vi "Get_DeviceInformation.vi"(8 "error in (no error)":errorcluster, 11 "Abstract_CCD in":refnum<class "Abstract_CCD.lvclass">) -> (0 "error out":errorcluster, 2 "Array":string[](array[string]), 3 "Abstract_CCD out":refnum<class "Abstract_CCD.lvclass">)   [LabVIEW 2020, in "Abstract_CCD.lvclass"]
uses:
  <instrlib>/Classes/CCD/Abstract_CCD/Abstract_CCD.lvclass
  <instrlib>/Classes/CCD/Abstract_CCD/FrameCombination.ctl
panel:
  out "FrameCombinationMethod":T1 items=["Sum"=1, "Average"=2]
  in  "Enum":enum16{"Not Defined", "Unlocked", "Locked"}(ring)
  in  "Trigger Mode":u16(ring) items=["Intern", "Extern"]
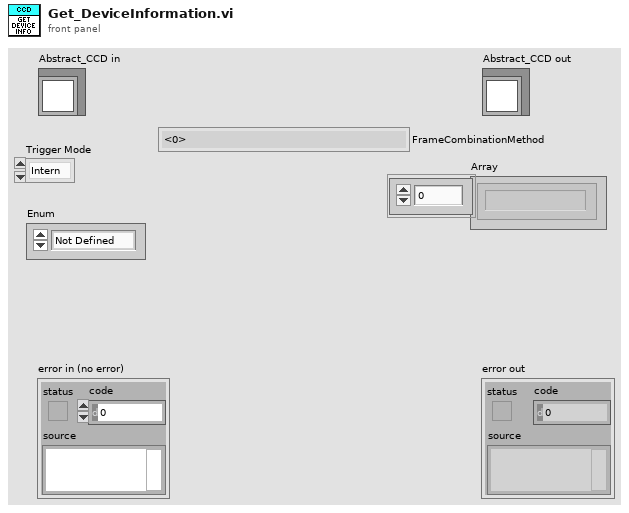
[diagram p1: front panel]
types:
  T1 = typedef "FrameCombination.ctl" = i32
  T2 = enum16{"Not Defined", "Unlocked", "Locked", "Not Reached"}
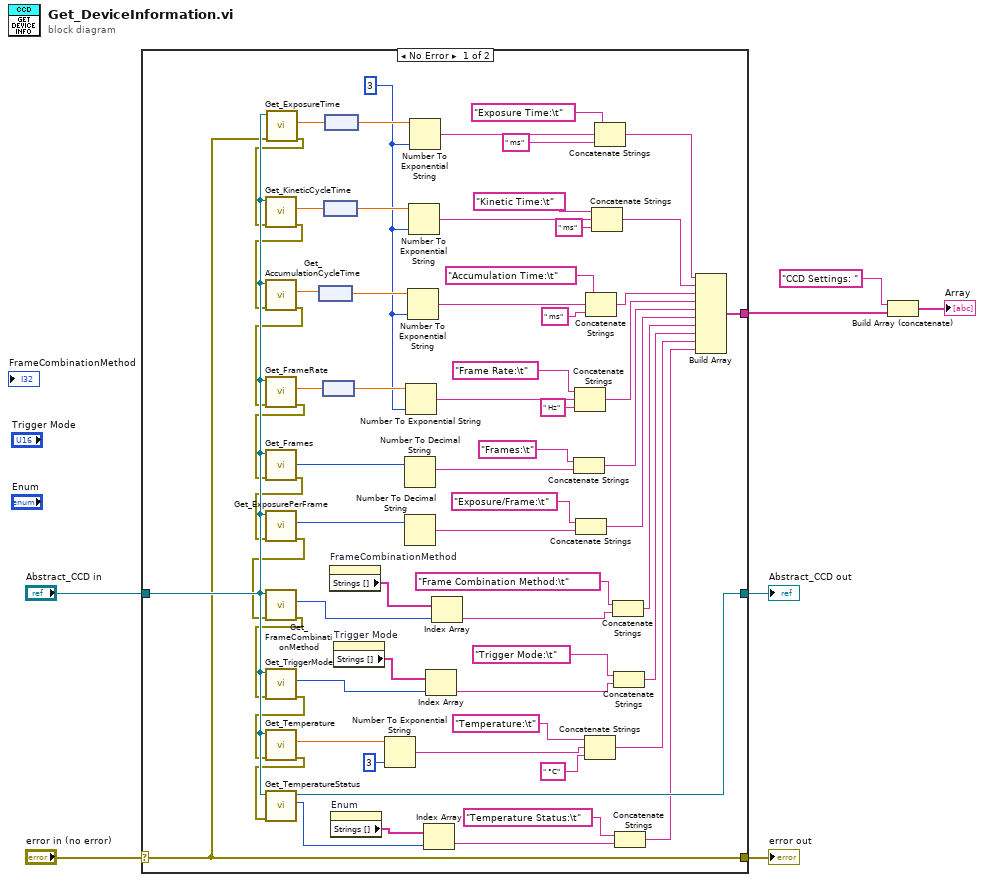
[diagram p0: block diagram]
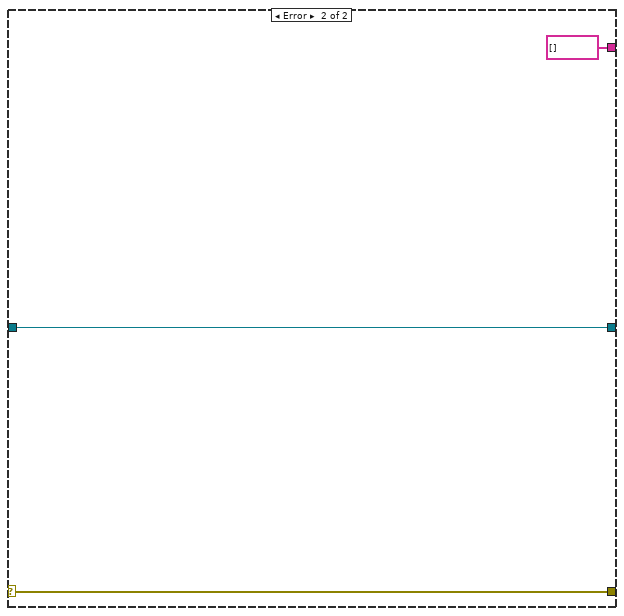
[diagram p2: hidden frame]
diagram:
  n1 = case shown="No Error" "error in (no error)" {
    selector: "error in (no error)" -> [w10 w77]
    tunnel: [w10 w77] -> w6
    tunnel: [w39 w76] -> w4
    tunnel: "Abstract_CCD in" -> [w74 w76]
    tunnel: [w19 string[] []] -> w2
    frame No Error {
      w56 = i16 3 ("precision (6)")
      n2 = call-dynamic "Get_ExposureTime.vi"("error in (no error)"=w10, "Abstract_CCD in"=w74) -> ("error out"=w18:errorcluster, "Exposure Time"=w73:dbl[unit])  [unwired: 7 in, 1 out]
      n3 = call-dynamic "Get_KineticCycleTime.vi"("error in (no error)"=w18, "Abstract_CCD in"=w74) -> ("error out"=w17:errorcluster, "Kinetic Cycle Time"=w68:dbl[unit])  [unwired: 7 in, 1 out]
      n4 = call-dynamic "Get_AccumulationCycleTime.vi"("error in (no error)"=w17, "Abstract_CCD in"=w74) -> ("error out"=w16:errorcluster, "Accumulation Cycle Time"=w63:dbl[unit])  [unwired: 7 in, 1 out]
      n5 = call-dynamic "Get_FrameRate.vi"("error in (no error)"=w16, "Abstract_CCD in"=w74) -> ("error out"=w15:errorcluster, "Frame Rate"=w58:dbl[unit])  [unwired: 7 in, 1 out]
      n6 = call-dynamic "Get_Frames.vi"("error in (no error)"=w15, "Abstract_CCD in"=w74) -> ("error out"=w14:errorcluster, "Numeric"=w52:i32)  [unwired: 7 in, 1 out]
      n7 = call-dynamic "Get_ExposurePerFrame.vi"("error in (no error)"=w14, "Abstract_CCD in"=w74) -> ("error out"=w13:errorcluster, "Exposure per Frame"=w49:i32)  [unwired: 7 in, 1 out]
      n8 = call-dynamic "Get_FrameCombinationMethod.vi"("error in (no error)"=w13, "Abstract_CCD in"=w74) -> ("error out"=w12:errorcluster, "FrameCombinationMethod"=w46:T1)  [unwired: 7 in, 1 out]
      n9 = call-dynamic "Get_TriggerMode.vi"("error in (no error)"=w12, "Abstract_CCD in"=w74) -> ("error out"=w11:errorcluster, "Trigger Mode"=w42:u16)  [unwired: 7 in, 1 out]
      n10 = call-dynamic "Get_Temperature.vi"("error in (no error)"=w11, "Abstract_CCD in"=w74) -> ("error out"=w9:errorcluster, "Temperature"=w38:dbl)  [unwired: 7 in, 1 out]
      n11 = call-dynamic "Get_TemperatureStatus.vi"("error in (no error)"=w9, "Abstract_CCD in"=w74) -> ("Enum"=w32:T2, "Abstract_CCD out"=w39:refnum<class "Abstract_CCD.lvclass">)  [unwired: 7 in, 1 out]
      n12 = node(w63) -> (w62:dbl)
      n13 = node(w58) -> (w57:dbl)
      n14 = node(w68) -> (w67:dbl)
      n15 = node(w73) -> (w72:dbl)
      n16 = property on="FrameCombinationMethod" class="Ring (strict)"() -> ("Strings []"=w8:string[])  [unwired: 2 in, 2 out]
      n17 = property on="Enum" class="Enum (strict)"() -> ("Strings []"=w33:string[])  [unwired: 2 in, 2 out]
      n18 = property on="Trigger Mode" class="Ring (strict)"() -> ("Strings []"=w43:string[])  [unwired: 2 in, 2 out]
      n19 = Number To Exponential String(number=w38, precision (6)=i16 3) -> (E-format string=w35:string)  [unwired: 2 in]
      n20 = Number To Decimal String(number=w52) -> (decimal integer string=w51:string)  [unwired: 1 in]
      n21 = Number To Decimal String(number=w49) -> (decimal integer string=w47:string)  [unwired: 1 in]
      n22 = Number To Exponential String(number=w57, precision (6)=w56) -> (E-format string=w55:string)  [unwired: 2 in]
      n23 = Number To Exponential String(number=w62, precision (6)=w56) -> (E-format string=w61:string)  [unwired: 2 in]
      n24 = Number To Exponential String(number=w67, precision (6)=w56) -> (E-format string=w65:string)  [unwired: 2 in]
      n25 = Number To Exponential String(number=w72, precision (6)=w56) -> (E-format string=w71:string)  [unwired: 2 in]
      n26 = Index Array(array=w33, index=w32) -> (element=w30:string)
      n27 = Index Array(array=w43, index=w42) -> (element=w40:string)
      n28 = Index Array(array=w8, index=w46) -> (element=w44:string)
      n29 = Concatenate Strings("Frames:\t", w51) -> (w25:string)
      n30 = Concatenate Strings("Frame Rate:\t", w55, " Hz" ("string")) -> (w26:string)
      n31 = Concatenate Strings("Exposure/Frame:\t", w47) -> (w24:string)
      n32 = Concatenate Strings("Temperature:\t", w35, " °C" ("string")) -> (w21:string)
      n33 = Concatenate Strings("Accumulation Time:\t", w61, " ms" ("string")) -> (w27:string)
      n34 = Concatenate Strings("Kinetic Time:\t", w65, " ms" ("string")) -> (w28:string)
      n35 = Concatenate Strings("Exposure Time:\t" ("string"), w71, " ms" ("string")) -> (w29:string)
      n36 = Concatenate Strings("Frame Combination Method:\t", w44) -> (w23:string)
      n37 = Concatenate Strings("Trigger Mode:\t", w40) -> (w22:string)
      n38 = Concatenate Strings("Temperature Status:\t", w30) -> (w20:string)
      n39 = Build Array(w29, w28, w27, w26, w25, w24, w23, w22, w21, w20) -> (w19:string[])
    }
    frame Error {
    }
  }
  "error out" <- w6
  "Abstract_CCD out" <- w4
  n40 = Build Array (concatenate)("CCD Settings: ", w2) -> (→"Array":string[])
